vi "Axsun GUI.vi"() -> ()   [LabVIEW 2018]
uses:
  serial sectioning OCT/Axsun/cluster_Axsun.ctl
  General/Controls/Queue Manager Actions.ctl
  General/Controls/MessagePacket.ctl
  Axsun action.ctl
panel:
  in  "stop":bool
  out "error out":errorcluster
  out "output cluster":T1
  in  "Source OFF":bool
  in  "Source ON":bool
  in  "Laser OFF":bool
  in  "Laser ON":bool
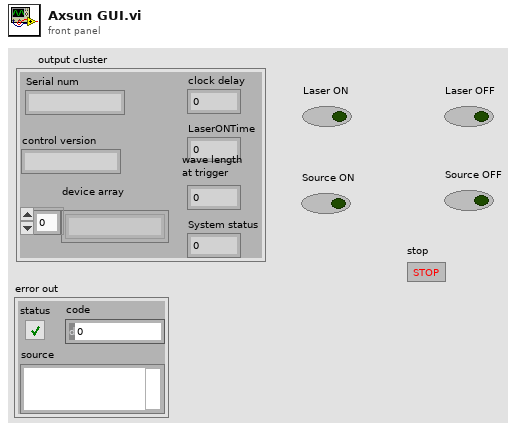
[diagram p1: front panel]
types:
  T1 = typedef "cluster_Axsun.ctl" = cluster{"device array":string[], "control version":string, "Serial num":string, "LaserONTime":i32, "wave length\nat trigger":dbl, "System status":dbl, "clock delay":u32}
  T2 = typedef "MessagePacket.ctl" = cluster{"Message":string, "Parameter":variant}
  T3 = typedef "Queue Manager Actions.ctl" = enum16{"Init", "Enqueue", "Enqueue All", "Preview Queue", "Dequeue", "Get Status", "Flush Queue", "Flush All Queues", "Release All Queues", "Release Queue", "Enqueue at Opposite End"}
  T4 = typedef "Axsun action.ctl" = enum16{"GetSystemStatus", "Clock delay", "GetLaserOnTime", "GetWaveLengthAtSweptTrigger", "Source current ON", "GetSerialNum", "GetControlVersion", "Laser ON", "Laser OFF", "Source current OFF", "Get laser handle", "Start Network Control Interface", "stop", "Create handle"}
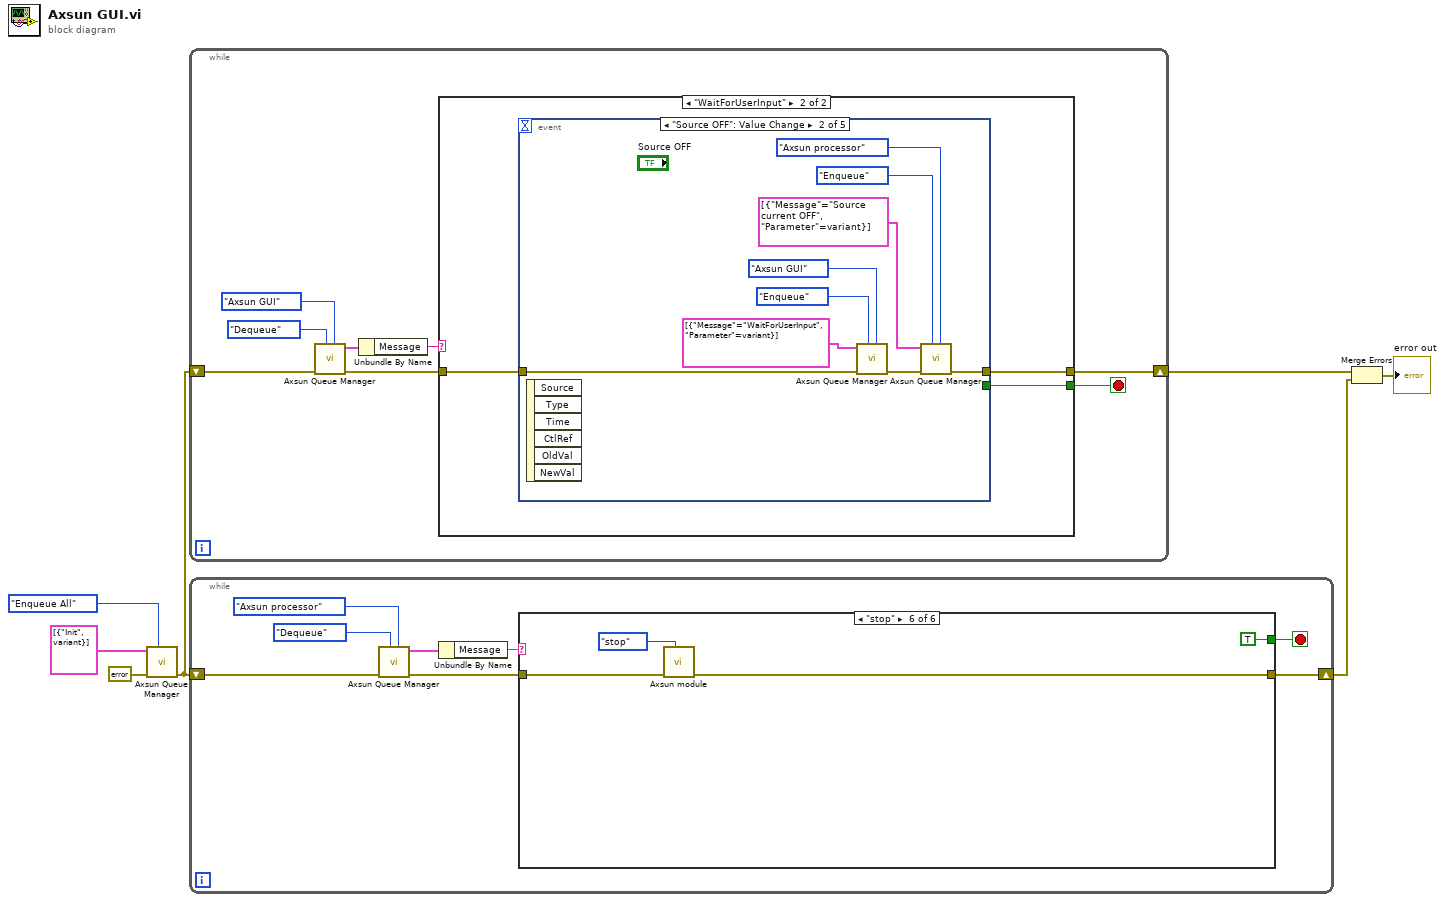
[diagram p0: block diagram]
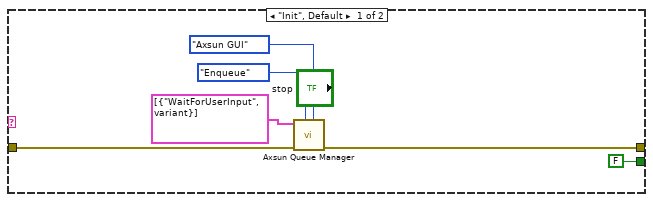
[diagram p2: hidden frame]
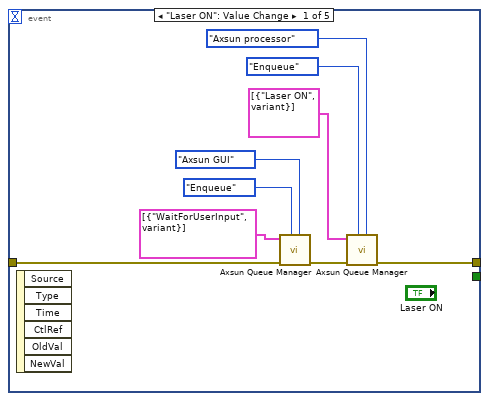
[diagram p3: hidden frame]
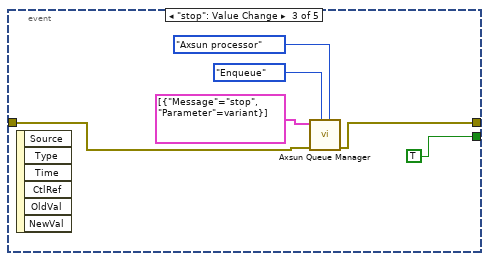
[diagram p4: hidden frame]
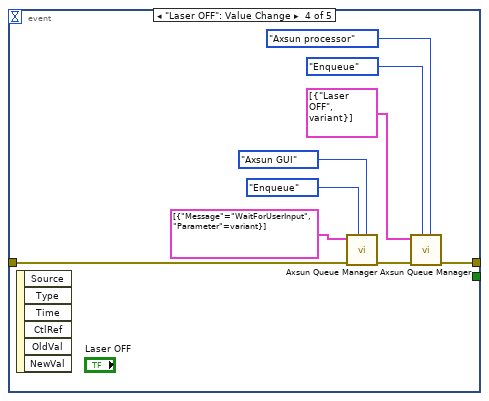
[diagram p5: hidden frame]
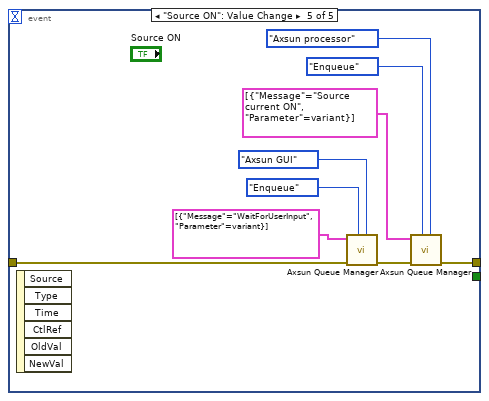
[diagram p6: hidden frame]
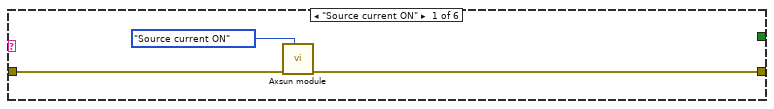
[diagram p7: hidden frame]
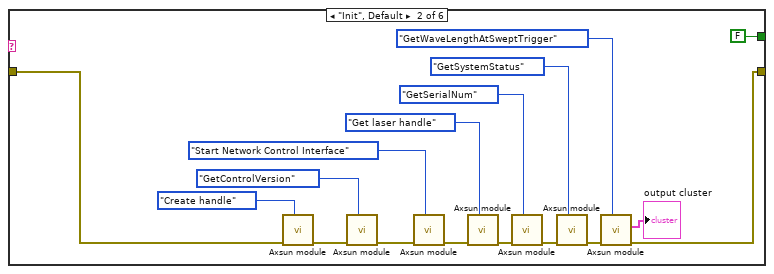
[diagram p8: hidden frame]
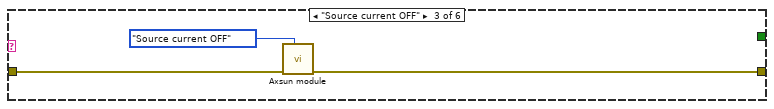
[diagram p9: hidden frame]
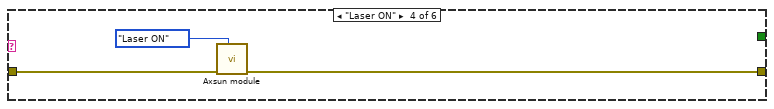
[diagram p10: hidden frame]
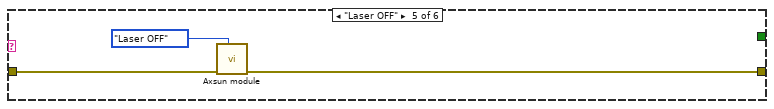
[diagram p11: hidden frame]
diagram:
  n1 = call "Axsun Queue Manager.vi"("Action"=Queue_Manager_Actions."Enqueue All", "Error In"=errorcluster {"status"=FALSE, "code"=0, "source"=""} ("error in (no error)"), "Message Packet Array"=T2[] [{"Message"="Init", "Parameter"=variant}]) -> ("Error Out"=w4:errorcluster)  [unwired: 5 in, 3 out]
  n2 = while {
    shift-right: [w10] -> w3
    shift-left: w4 -> [w12]
    stop <- w9 stop-if-true
    n3 = call "Axsun Queue Manager.vi"("queue name"=enum16{"Axsun processor", "Axsun GUI"}."Axsun GUI", "Action"=Queue_Manager_Actions."Dequeue", "Error In"=w12) -> ("Error Out"=w11:errorcluster, "Message Packet [Out]"=w13:T2)  [unwired: 5 in, 2 out]
    n4 = Unbundle By Name(w13) -> ("Message"=w8:string)
    n5 = case shown="\"WaitForUserInput\"" w8 {
      tunnel: w11 -> [w21 w24]
      tunnel: [w20 w23] -> w10
      tunnel: [FALSE w22] -> w9
      frame "Init", Default {
        n6 = call "Axsun Queue Manager.vi"("queue name"=enum16{"Axsun processor", "Axsun GUI"}."Axsun GUI", "Action"=Queue_Manager_Actions."Enqueue", "Error In"=w21, "Message Packet Array"=T2[] [{"Message"="WaitForUserInput", "Parameter"=variant}]) -> ("Error Out"=w20:errorcluster)  [unwired: 4 in, 3 out]
      }
      frame "WaitForUserInput" {
        n7 = event shown="[1] \"Source OFF\": Value Change" {
          selector: _ -> [_ _ _ _ _]
          dyn-events: _ -> [_ _ _ _ _]
          timeout: _ -> [_ _ _ _ _]
          tunnel: w24 -> [w33 w35 w45 w51 w60]
          tunnel: [w31 w34 w44 w49 w58] -> w23
          tunnel: [_ _ TRUE _ _] -> w22
          event "Laser ON": Value Change {
            n8 = event-data() -> ()  [unwired: 1 in, 6 out]
            n9 = call "Axsun Queue Manager.vi"("queue name"=enum16{"Axsun processor", "Axsun GUI"}."Axsun GUI", "Action"=Queue_Manager_Actions."Enqueue", "Error In"=w33, "Message Packet Array"=T2[] [{"Message"="WaitForUserInput", "Parameter"=variant}]) -> ("Error Out"=w32:errorcluster)  [unwired: 4 in, 3 out]
            n10 = call "Axsun Queue Manager.vi"("queue name"=enum16{"Axsun processor", "Axsun GUI"}."Axsun processor", "Action"=Queue_Manager_Actions."Enqueue", "Error In"=w32, "Message Packet Array"=T2[] [{"Message"="Laser ON", "Parameter"=variant}]) -> ("Error Out"=w31:errorcluster)  [unwired: 4 in, 3 out]
          }
          event "Source OFF": Value Change {
            n11 = event-data() -> ()  [unwired: 1 in, 6 out]
            n12 = call "Axsun Queue Manager.vi"("queue name"=enum16{"Axsun processor", "Axsun GUI"}."Axsun GUI", "Action"=Queue_Manager_Actions."Enqueue", "Error In"=w35, "Message Packet Array"=T2[] [{"Message"="WaitForUserInput", "Parameter"=variant}] ("Message Packet [In]")) -> ("Error Out"=w42:errorcluster)  [unwired: 4 in, 3 out]
            n13 = call "Axsun Queue Manager.vi"("queue name"=enum16{"Axsun processor", "Axsun GUI"}."Axsun processor", "Action"=Queue_Manager_Actions."Enqueue", "Error In"=w42, "Message Packet Array"=T2[] [{"Message"="Source current OFF", "Parameter"=variant}]) -> ("Error Out"=w34:errorcluster)  [unwired: 4 in, 3 out]
          }
          event "stop": Value Change {
            n14 = event-data() -> ()  [unwired: 1 in, 6 out]
            n15 = call "Axsun Queue Manager.vi"("queue name"=enum16{"Axsun processor", "Axsun GUI"}."Axsun processor", "Action"=Queue_Manager_Actions."Enqueue", "Error In"=w45, "Message Packet Array"=T2[] [{"Message"="stop", "Parameter"=variant}]) -> ("Error Out"=w44:errorcluster)  [unwired: 4 in, 3 out]
          }
          event "Laser OFF": Value Change {
            n16 = event-data() -> ()  [unwired: 1 in, 6 out]
            n17 = call "Axsun Queue Manager.vi"("queue name"=enum16{"Axsun processor", "Axsun GUI"}."Axsun GUI", "Action"=Queue_Manager_Actions."Enqueue", "Error In"=w51, "Message Packet Array"=T2[] [{"Message"="WaitForUserInput", "Parameter"=variant}] ("Message Packet [In]")) -> ("Error Out"=w57:errorcluster)  [unwired: 4 in, 3 out]
            n18 = call "Axsun Queue Manager.vi"("queue name"=enum16{"Axsun processor", "Axsun GUI"}."Axsun processor", "Action"=Queue_Manager_Actions."Enqueue", "Error In"=w57, "Message Packet Array"=T2[] [{"Message"="Laser OFF", "Parameter"=variant}]) -> ("Error Out"=w49:errorcluster)  [unwired: 4 in, 3 out]
          }
          event "Source ON": Value Change {
            n19 = event-data() -> ()  [unwired: 1 in, 6 out]
            n20 = call "Axsun Queue Manager.vi"("queue name"=enum16{"Axsun processor", "Axsun GUI"}."Axsun GUI", "Action"=Queue_Manager_Actions."Enqueue", "Error In"=w60, "Message Packet Array"=T2[] [{"Message"="WaitForUserInput", "Parameter"=variant}] ("Message Packet [In]")) -> ("Error Out"=w66:errorcluster)  [unwired: 4 in, 3 out]
            n21 = call "Axsun Queue Manager.vi"("queue name"=enum16{"Axsun processor", "Axsun GUI"}."Axsun processor", "Action"=Queue_Manager_Actions."Enqueue", "Error In"=w66, "Message Packet Array"=T2[] [{"Message"="Source current ON", "Parameter"=variant}]) -> ("Error Out"=w58:errorcluster)  [unwired: 4 in, 3 out]
          }
        }
      }
    }
  }
  n22 = while {
    shift-right: [w68] -> w2
    shift-left: w4 -> [w74]
    stop <- w67 stop-if-true
    n23 = call "Axsun Queue Manager.vi"("queue name"=enum16{"Axsun processor", "Axsun GUI"}."Axsun processor", "Action"=Queue_Manager_Actions."Dequeue", "Error In"=w74) -> ("Error Out"=w73:errorcluster, "Message Packet [Out]"=w70:T2)  [unwired: 5 in, 2 out]
    n24 = Unbundle By Name(w70) -> ("Message"=w69:string)
    n25 = case shown="\"stop\"" w69 {
      tunnel: w73 -> [w77 w81 w96 w99 w102 w106]
      tunnel: [w76 w80 w95 w98 w101 w105] -> w68
      tunnel: [_ FALSE _ _ _ TRUE] -> w67
      frame "Source current ON" {
        n26 = call "Axsun module.vi"("Action"=Axsun_action."Source current ON", "error in (no error)"=w77) -> ("error out"=w76:errorcluster)  [unwired: 8 in, 1 out]
      }
      frame "Init", Default {
        n27 = call "Axsun module.vi"("Action"=Axsun_action."Create handle", "error in (no error)"=w81) -> ("error out"=w93:errorcluster)  [unwired: 8 in, 1 out]
        n28 = call "Axsun module.vi"("Action"=Axsun_action."GetControlVersion", "error in (no error)"=w93) -> ("error out"=w92:errorcluster)  [unwired: 8 in, 1 out]
        n29 = call "Axsun module.vi"("Action"=Axsun_action."Start Network Control Interface", "error in (no error)"=w92) -> ("error out"=w91:errorcluster)  [unwired: 8 in, 1 out]
        n30 = call "Axsun module.vi"("Action"=Axsun_action."Get laser handle", "error in (no error)"=w91) -> ("error out"=w90:errorcluster)  [unwired: 8 in, 1 out]
        n31 = call "Axsun module.vi"("Action"=Axsun_action."GetSerialNum", "error in (no error)"=w90) -> ("error out"=w89:errorcluster)  [unwired: 8 in, 1 out]
        n32 = call "Axsun module.vi"("Action"=Axsun_action."GetSystemStatus", "error in (no error)"=w89) -> ("error out"=w88:errorcluster)  [unwired: 8 in, 1 out]
        n33 = call "Axsun module.vi"("Action"=Axsun_action."GetWaveLengthAtSweptTrigger", "error in (no error)"=w88) -> ("error out"=w80:errorcluster, "output cluster"=→"output cluster":T1)  [unwired: 8 in]
      }
      frame "Source current OFF" {
        n34 = call "Axsun module.vi"("Action"=Axsun_action."Source current OFF", "error in (no error)"=w96) -> ("error out"=w95:errorcluster)  [unwired: 8 in, 1 out]
      }
      frame "Laser ON" {
        n35 = call "Axsun module.vi"("Action"=Axsun_action."Laser ON", "error in (no error)"=w99) -> ("error out"=w98:errorcluster)  [unwired: 8 in, 1 out]
      }
      frame "Laser OFF" {
        n36 = call "Axsun module.vi"("Action"=Axsun_action."Laser OFF", "error in (no error)"=w102) -> ("error out"=w101:errorcluster)  [unwired: 8 in, 1 out]
      }
      frame "stop" {
        n37 = call "Axsun module.vi"("Action"=Axsun_action."stop", "error in (no error)"=w106) -> ("error out"=w105:errorcluster)  [unwired: 8 in, 1 out]
      }
    }
  }
  n38 = Merge Errors(w3, w2) -> (→"error out":errorcluster)
